vi "_QMH_Init.vi"(7 "max queue size (-1, unlimited)":i32=20, 8 "error in (no error)":errorcluster, 10 "name (unnamed)":string) -> (0 "error out":errorcluster, 3 "QMH out":refnum<class "QMH.lvclass">)   [LabVIEW 2018, in "QMH.lvclass"]
uses:
  QMH.lvclass
  QMH.lvclass/QMH.ctl
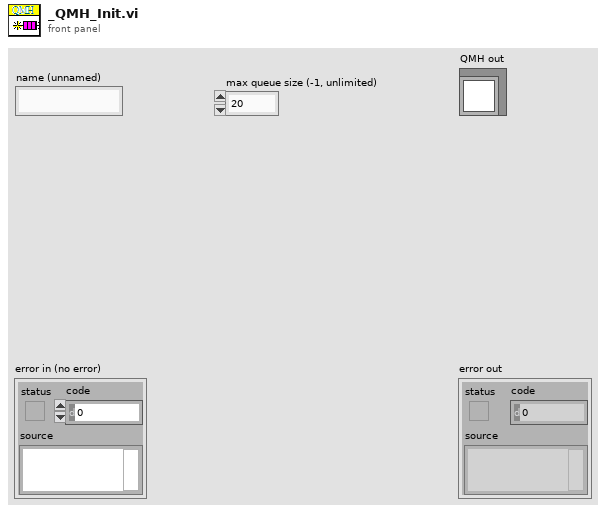
[diagram p1: front panel]
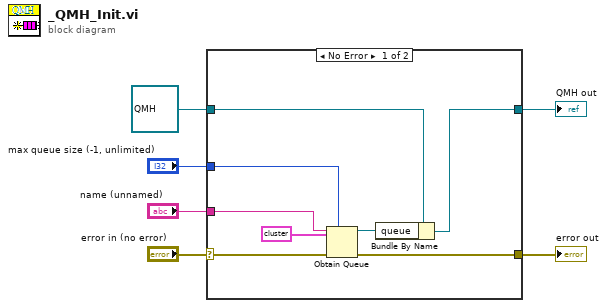
[diagram p0: block diagram]
diagram:
  n1 = case shown="No Error" "error in (no error)" {
    selector: "error in (no error)" -> [w8 w16]
    tunnel: [w7 w16] -> w5
    tunnel: [w13 w15] -> w3
    tunnel: refnum<class "QMH.lvclass"> refnum ("QMH in") -> [w14 w15]
    tunnel: "name (unnamed)" -> [w10 _]
    tunnel: "max queue size (-1, unlimited)" -> [w9 _]
    frame No Error {
      n2 = Obtain Queue(max queue size (-1, unlimited)=w9, name (unnamed)=w10, element data type=cluster{"Data":variant, "Msg":string} {"Data"=variant, "Msg"=""}, error in (no error)=w8) -> (queue out=w11:refnum<queue>, error out=w7:errorcluster)  [unwired: 1 in, 1 out]
      n3 = Bundle By Name(cluster=w14, "queue"=w11) -> (w13:refnum<class "QMH.lvclass">)
    }
    frame Error {
    }
  }
  "error out" <- w5
  "QMH out" <- w3
